vi "sendValue.vi"(8 "error in (no error)":errorcluster, 10 "data":variant, 11 "enterControl in":refnum<class "enterControl.lvclass">) -> (0 "error out":errorcluster, 2 "function return":i32, 3 "enterControl out":refnum<class "enterControl.lvclass">)   [LabVIEW 2016, in "SALLV_EXA_Messaging.lvlib" / "enterControl.lvclass"]
uses:
  enterControl.lvclass
  ts_sallv_MtAtElectrometer/DataTypes/command_disable.ctl
  enterControl.lvclass/enterControl.ctl
  ts_sallv_MtAtElectrometer/SALLV_MtAtElectrometer.lvlib
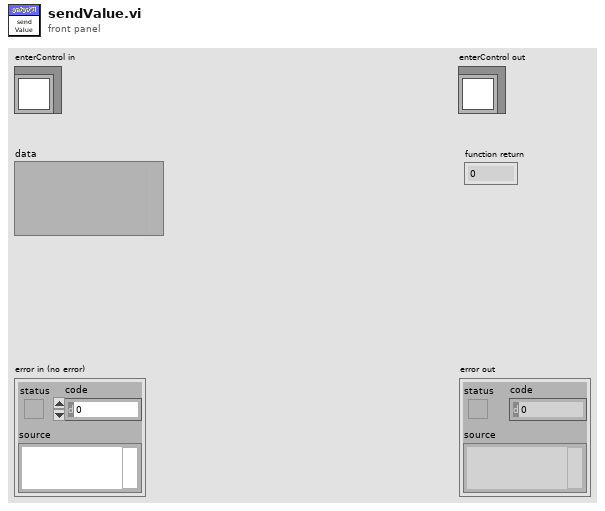
[diagram p1: front panel]
types:
  T1 = typedef "SALLV_MtAtElectrometer.lvlib/command_disable.ctl" = cluster{"value":bool}
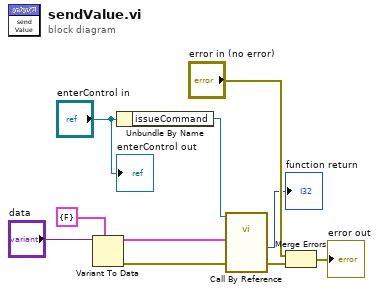
[diagram p0: block diagram]
diagram:
  n1 = Variant To Data(type=T1 {"value"=FALSE} ("command_enterControl_Ctl"), Variant="data") -> (data=w2:T1, error out=w1:errorcluster)  [unwired: 1 in]
  n2 = Unbundle By Name("enterControl in") -> ("issueCommand"=w7:refnum<vi>)
  n3 = call-by-ref "?"(reference=w7, "error in (no error)"=w1, "command_disable_Ctl"=w2) -> ("error out"=w8:errorcluster, "function return"=→"function return":i32)  [unwired: 8 in, 3 out]
  n4 = Merge Errors("error in (no error)", w8) -> (→"error out":errorcluster)
  "enterControl out" <- "enterControl in"
